vi "encodeImage.vi"(8 "error in (no error)":errorcluster, 10 "ImageData":T1, 11 "CameraNetworkClient in":refnum<class "CameraNetworkServer.lvclass">) -> (0 "error out":errorcluster, 2 "MessageString":string, 3 "CameraNetworkClient out":refnum<class "CameraNetworkServer.lvclass">)   [LabVIEW 2011, in "Hardware.lvlib" / "HWControllers.lvlib" / "CameraNetworkServer.lvclass"]
uses:
  CameraNetworkServer.lvclass
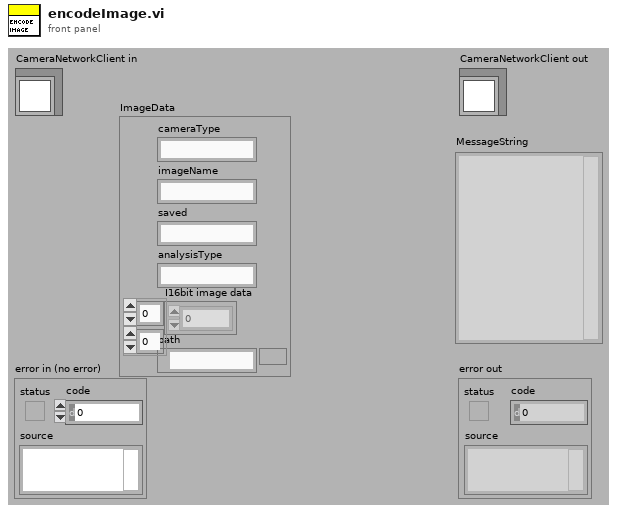
[diagram p1: front panel]
types:
  T1 = cluster{"cameraType":string, "imageName":string, "saved":string, "analysisType":string, "I16bit image data":i16[][], "path":path}
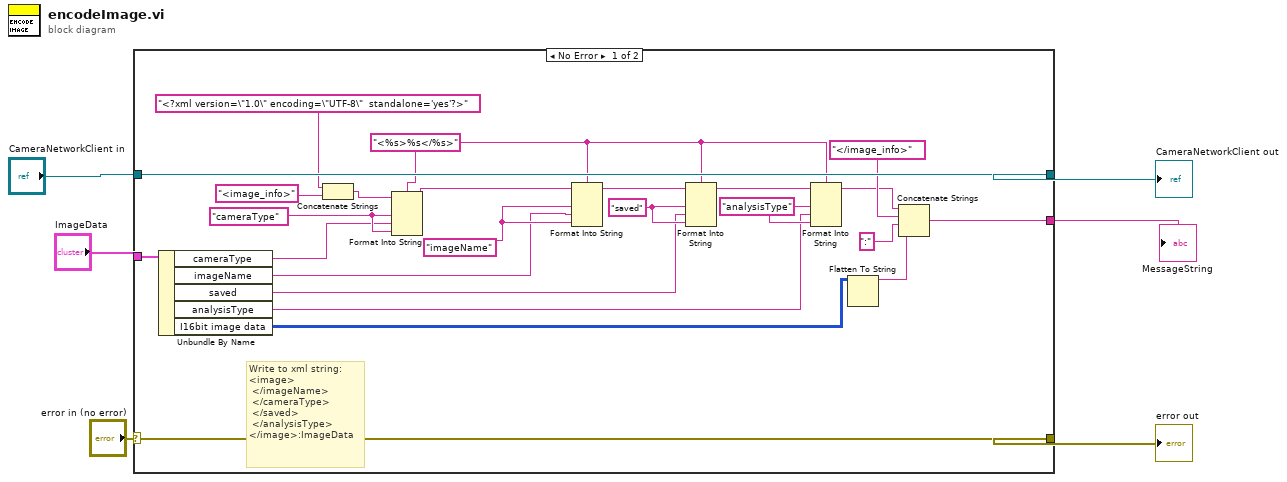
[diagram p0: block diagram]
diagram:
  n1 = case shown="No Error" "error in (no error)" {
    selector: "error in (no error)" -> [w7 w32]
    tunnel: [w7 w32] -> w5
    tunnel: [w30 w31] -> w3
    tunnel: "CameraNetworkClient in" -> [w30 w31]
    tunnel: "ImageData" -> [w18 _]
    tunnel: [w19 _] -> w1
    frame No Error {
      w14 = "analysisType"
      w24 = "saved"
      w12 = "<%s>%s</%s>"
      w28 = "imageName" ("Key")
      w29 = "cameraType"
      # "Write to xml string:\n<image>\n </imageName>\n </cameraType>\n </saved>\n </analysisType>\n</image>:ImageData"
      n2 = Unbundle By Name(w18) -> ("cameraType"=w17:string, "imageName"=w16:string, "saved"=w15:string, "analysisType"=w11:string, "I16bit image data"=w8:i16[][])
      n3 = Concatenate Strings("<?xml version=\"1.0\" encoding=\"UTF-8\"  standalone='yes'?>", "<image_info>") -> (w22:string)
      n4 = Format Into String(format string=w12, initial string=w22, w29, w17, w29) -> (resulting string=w26:string)  [unwired: 1 in, 1 out]
      n5 = Format Into String(format string=w12, initial string=w26, w28, w16, w28) -> (resulting string=w25:string)  [unwired: 1 in, 1 out]
      n6 = Format Into String(format string=w12, initial string=w25, w24, w15, w24) -> (resulting string=w13:string)  [unwired: 1 in, 1 out]
      n7 = Format Into String(format string=w12, initial string=w13, w14, w11, w14) -> (resulting string=w10:string)  [unwired: 1 in, 1 out]
      n8 = Flatten To String(anything=w8) -> (data string=w9:string)  [unwired: 3 in, 2 out]
      n9 = Concatenate Strings(w10, "</image_info>", ":", w9) -> (w19:string)
    }
    frame Error {
    }
  }
  "error out" <- w5
  "CameraNetworkClient out" <- w3
  "MessageString" <- w1
